vi "const_bias_conductance.vi"() -> ()   [LabVIEW 2010]
uses:
  <vilib>/Utility/file.llb/Write To Spreadsheet File (DBL).vi
  <userlib>/Nanonis Prog Interface V5/Nanonis Prog Interface.lvlib
panel:
  in  "Bias (V)":sgl format="%_5p"
  in  "Feedback?":bool=TRUE
  in  "Settling Time between gate":u32=5
  in  "Wait Time between AVG":i32=1
  out "Input 2 (V)":sgl
  out "XY Graph":cluster{dbl[], dbl[]}(graph)
  in  "Averages":i32=5
  out "Current Gate Voltage (V)":dbl
  in  "Stop":bool
  in  "Increment Gate (V)":dbl
  in  "End Gate (V)":dbl
  in  "Start Gate (V)":dbl
  in  "Filename":string
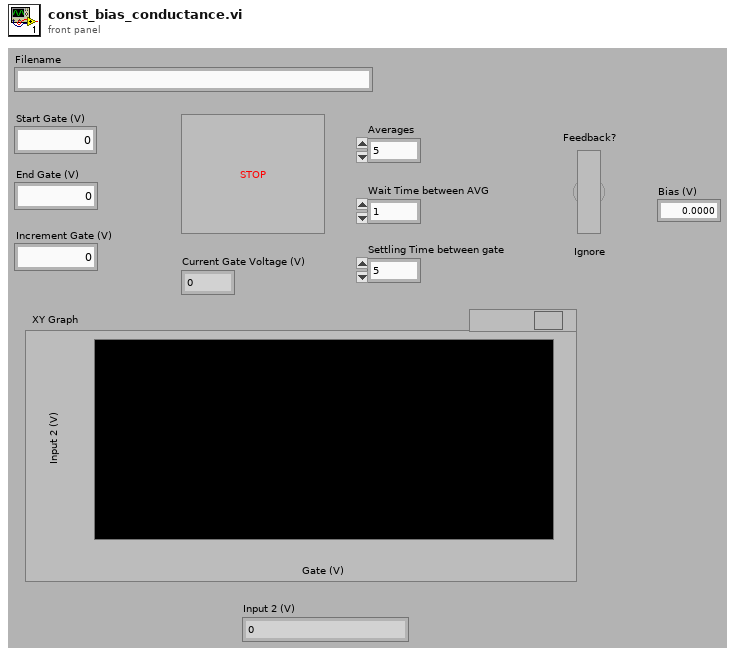
[diagram p1: front panel]
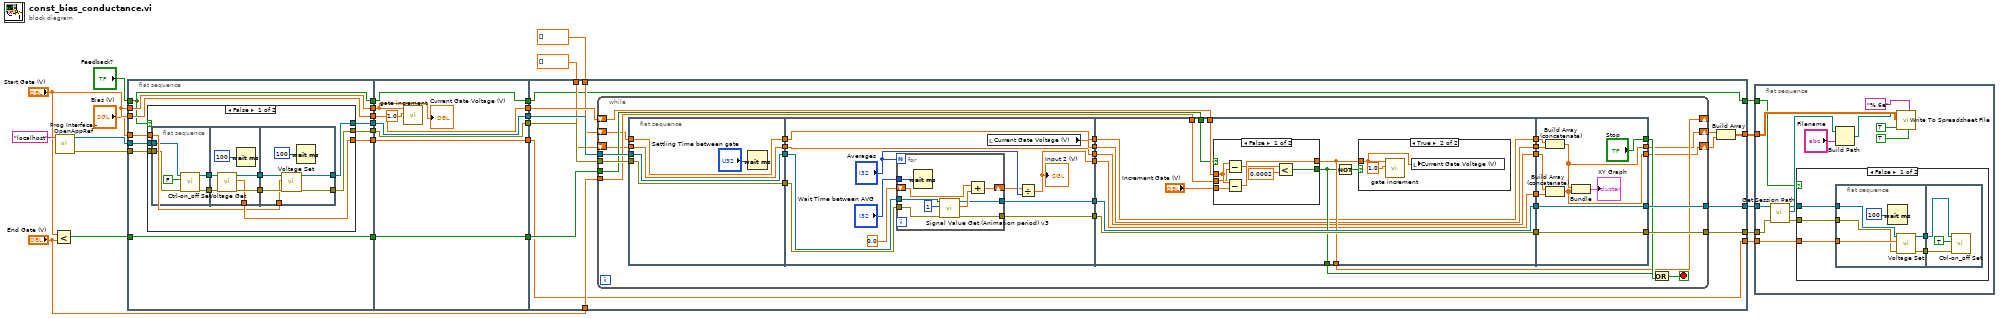
[diagram p0: block diagram]
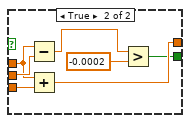
[diagram p4: hidden frame]
diagram:
  n1 = Less?(x="Start Gate (V)", y="End Gate (V)") -> (x < y?=w25:bool)
  n2 = call <userlib>:"Prog Interface - OpenAppRef.vi"("Machine name (local machine IP)"="localhost" ("machine name (localhost)")) -> ("Error out"=w17:errorcluster, "Application reference"=w18:refnum<vi>)  [unwired: 5 in]
  n3 = flat-sequence {
    tunnel: "Start Gate (V)" -> [w36]
    tunnel: "Start Gate (V)" -> [w37]
    tunnel: w25 -> [w38]
    tunnel: w18 -> [w35]
    tunnel: w17 -> [w32]
    tunnel: [w38] -> w13
    tunnel: [w37] -> w12
    tunnel: [w36] -> w11
    tunnel: "Feedback?" -> [w31]
    tunnel: [w34] -> w9
    tunnel: [w33] -> w8
    tunnel: [w31] -> w7
    tunnel: [w30] -> w4
    tunnel: "Bias (V)" -> [w29]
    tunnel: [w76] -> w24
    tunnel: [w75] -> w23
    tunnel: [w74] -> w22
    tunnel: [w73] -> w21
    tunnel: w13 -> [w74]
    tunnel: w12 -> [w73]
    tunnel: w11 -> [w71]
    tunnel: w9 -> [w75]
    tunnel: w8 -> [w76]
    tunnel: w7 -> [w70]
    tunnel: [w70] -> w6
    tunnel: w4 -> [w69]
    tunnel: [w69] -> w3
    tunnel: [w88] -> w27
    tunnel: [w87] -> w26
    tunnel: w24 -> [w90]
    tunnel: w23 -> [w89]
    tunnel: w22 -> [w86]
    tunnel: w21 -> [w85]
    tunnel: "End Gate (V)" -> [w84]
    tunnel: [w81] -> w16
    tunnel: dbl[] [] -> [w80]
    tunnel: dbl[] [] -> [w79]
    tunnel: w6 -> [w78]
    tunnel: [w78] -> w5
    tunnel: w3 -> [w77]
    tunnel: [w77] -> w2
    frame #0 {
      n4 = case shown="False" w31 {
        tunnel: w35 -> [w48 w68]
        tunnel: [w41 w68] -> w34
        tunnel: [w40 w67] -> w33
        tunnel: w32 -> [w47 w67]
        tunnel: [w42 w66] -> w30
        tunnel: w29 -> [w39 w66]
        frame False {
          n5 = flat-sequence {
            tunnel: w48 -> [w53]
            tunnel: w47 -> [w52]
            tunnel: [w50] -> w46
            tunnel: [w49] -> w45
            tunnel: w46 -> [w59]
            tunnel: w45 -> [w58]
            tunnel: [w57] -> w44
            tunnel: [w56] -> w43
            tunnel: [w55] -> w42
            tunnel: w44 -> [w65]
            tunnel: w43 -> [w64]
            tunnel: [w62] -> w41
            tunnel: [w61] -> w40
            tunnel: w39 -> [w60]
            frame #0 {
              n6 = call <userlib>:"Ctrl-on_off Set.vi"("error in (no error)"=w52, "Z Controller ON/OFF"=FALSE, "Application ref in"=w53) -> ("error out"=w49:errorcluster, "Application ref out"=w50:refnum<vi>)  [unwired: 7 in]
            }
            frame #1 {
              n7 = call <userlib>:"Voltage Get.vi"("error in (no error)"=w58, "Application ref in"=w59) -> ("error out"=w57:errorcluster, "Bias (V)"=w55:sgl, "Application ref out"=w56:refnum<vi>)  [unwired: 7 in]
              n8 = Wait (ms)(milliseconds to wait=u32 100) -> ()  [unwired: 1 out]
            }
            frame #2 {
              n9 = call <userlib>:"Voltage Set.vi"("Error in (no error)"=w65, "Bias (V)"=w60, "Application ref in"=w64) -> ("Error out"=w61:errorcluster, "Application ref out"=w62:refnum<vi>)  [unwired: 7 in]
              n10 = Wait (ms)(milliseconds to wait=u32 100) -> ()  [unwired: 1 out]
            }
          }
        }
        frame True {
        }
      }
    }
    frame #1 {
      n11 = call "gate increment.vi"("Increment"=1.0, "Gate Voltage"=w71) -> ()  [unwired: 8 in, 2 out]
      "Current Gate Voltage (V)" <- w71
    }
    frame #2 {
      n12 = while {
        tunnel: w90 -> [w121]
        tunnel: w89 -> [w120]
        tunnel: [w119] -> w88
        tunnel: [w118] -> w87
        tunnel: w86 -> [w107]
        shift-right: [w111] -> _
        shift-left: w85 -> [w109]
        tunnel: w84 -> [w108]
        shift-right: [w101] -> w83
        shift-left: w80 -> [w100]
        shift-right: [w98] -> w82
        shift-left: w79 -> [w93]
        stop <- w112 stop-if-true
        n13 = flat-sequence {
          tunnel: w120 -> [w125]
          tunnel: w121 -> [w126]
          tunnel: [w126] -> w115
          tunnel: [w125] -> w114
          tunnel: w100 -> [w123]
          tunnel: w93 -> [w124]
          tunnel: [w124] -> w94
          tunnel: [w123] -> w92
          tunnel: w115 -> [w138]
          tunnel: w114 -> [w134]
          tunnel: [w133] -> w106
          tunnel: [w132] -> w105
          tunnel: [w131] -> w104
          tunnel: [w129] -> w97
          tunnel: [w130] -> w96
          tunnel: w94 -> [w129]
          tunnel: w92 -> [w128]
          tunnel: [w128] -> w91
          tunnel: [w160] -> w117
          tunnel: [w159] -> w116
          tunnel: [w158] -> w111
          tunnel: [w157] -> w110
          tunnel: w109 -> [w156]
          tunnel: w108 -> [w154]
          tunnel: w107 -> [w153]
          tunnel: w106 -> [w159]
          tunnel: w105 -> [w160]
          tunnel: w104 -> [w151]
          tunnel: [w151] -> w103
          tunnel: [w150] -> w102
          tunnel: [w149] -> w99
          tunnel: w97 -> [w149]
          tunnel: w96 -> [w148]
          tunnel: [w148] -> w95
          tunnel: w91 -> [w150]
          tunnel: [w185] -> w119
          tunnel: [w186] -> w118
          tunnel: w117 -> [w186]
          tunnel: w116 -> [w185]
          tunnel: ["Stop"] -> w113
          tunnel: [w178] -> w101
          tunnel: w103 -> [w183]
          tunnel: w102 -> [w182]
          tunnel: w99 -> [w181]
          tunnel: [w177] -> w98
          tunnel: w95 -> [w180]
          frame #0 {
            n14 = Wait (ms)(milliseconds to wait="Settling Time between gate") -> ()  [unwired: 1 out]
          }
          frame #1 {
            n15 = for {
              N: "Averages" -> [_]
              tunnel: w134 -> [w146]
              tunnel: w138 -> [w145]
              shift-right: [w142] -> w136
              shift-left: sgl 0.0 -> [w143]
              tunnel: [w141] -> w133
              tunnel: [w140] -> w132
              tunnel: "Wait Time between AVG" -> [w139]
              n16 = Wait (ms)(milliseconds to wait=w139) -> ()  [unwired: 1 out]
              n17 = call <userlib>:"Signal Value Get (Animation period) v3.vi"("error in (no error)"=w145, "Signal index (0-127)"=i8 1, "Application ref in"=w146) -> ("error out"=w140:errorcluster, "Signal value"=w144:sgl, "Application ref out"=w141:refnum<vi>)  [unwired: 5 in]
              n18 = Add(x=w143, y=w144) -> (x+y=w142:sgl)
            }
            n19 = local read "Current Gate Voltage (V)"() -> (w131:dbl)
            n20 = Divide(x=w136, y="Averages") -> (x/y=w130:sgl)
            "Input 2 (V)" <- w130
          }
          frame #2 {
            n21 = case shown="False" w153 {
              tunnel: w156 -> [w165 w171]
              tunnel: "Increment Gate (V)" -> [w166 w174]
              tunnel: [w167 w173] -> w158
              tunnel: w154 -> [w164 w172]
              tunnel: [w162 w170] -> w157
              frame False {
                n22 = Subtract(x=w165, y=w164) -> (x-y=w163:dbl)
                n23 = Subtract(x=w165, y=w166) -> (x-y=w167:dbl)
                n24 = Less?(x=w163, y=0.0002) -> (x < y?=w162:bool)
              }
              frame True {
                n25 = Subtract(x=w171, y=w172) -> (x-y=w169:dbl)
                n26 = Add(x=w171, y=w174) -> (x+y=w173:dbl)
                n27 = Greater?(x=w169, y=-0.0002) -> (0:w170:bool)
              }
            }
            n28 = Not(x=w157) -> (.not. x?=w152:bool)
            n29 = case shown="True" w152 {
              tunnel: w158 -> [_ w175]
              frame False {
              }
              frame True {
                n30 = call "gate increment.vi"("Increment"=1.0, "Gate Voltage"=w175) -> ()  [unwired: 8 in, 2 out]
                n31 = local write "Current Gate Voltage (V)"(w175) -> ()
              }
            }
          }
          frame #3 {
            n32 = Build Array (concatenate)(w182, w183) -> (w178:dbl[])
            n33 = Build Array (concatenate)(w181, w180) -> (w177:dbl[])
            n34 = Bundle(w178, w177) -> (→"XY Graph":cluster{dbl[], dbl[]})  [unwired: 1 in]
          }
        }
        n35 = Or(x=w110, y=w113) -> (x .or. y?=w112:bool)
      }
      n36 = Build Array(w83, w82) -> (w81:dbl[][])
    }
  }
  n37 = flat-sequence {
    tunnel: w27 -> [w196]
    tunnel: w26 -> [w195]
    tunnel: w16 -> [w197]
    tunnel: w5 -> [w190]
    tunnel: w2 -> [w189]
    frame #0 {
      n38 = call <userlib>:"Get Session Path.vi"("error in (no error)"=w195, "Application ref in"=w196) -> ("error out"=w187:errorcluster, "Session path"=w192:path, "Application ref out"=w188:refnum<vi>)  [unwired: 7 in]
      n39 = case shown="False" w190 {
        tunnel: w189 -> [w204 _]
        tunnel: w188 -> [w203 _]
        tunnel: w187 -> [w202 _]
        frame False {
          n40 = flat-sequence {
            tunnel: w204 -> [w210]
            tunnel: w203 -> [w209]
            tunnel: w202 -> [w208]
            tunnel: [w207] -> w201
            tunnel: [w206] -> w200
            tunnel: w201 -> [w213]
            tunnel: w200 -> [w212]
            frame #0 {
              n41 = Wait (ms)(milliseconds to wait=u32 100) -> ()  [unwired: 1 out]
              n42 = call <userlib>:"Voltage Set.vi"("Error in (no error)"=w208, "Bias (V)"=w210, "Application ref in"=w209) -> ("Error out"=w206:errorcluster, "Application ref out"=w207:refnum<vi>)  [unwired: 7 in]
            }
            frame #1 {
              n43 = call <userlib>:"Ctrl-on_off Set.vi"("error in (no error)"=w212, "Z Controller ON/OFF"=TRUE, "Application ref in"=w213) -> ()  [unwired: 7 in, 2 out]
            }
          }
        }
        frame True {
        }
      }
      n44 = Build Path(base path=w192, name or relative path="Filename") -> (appended path=w194:path)
      n45 = call-poly <vilib>:"Write To Spreadsheet File.vi"("transpose? (no:F)"=TRUE ("append to file? (new file:F)"), "format (%.3f)"="%.6e", "append to file? (new file:F)"=TRUE, "2D data"=w197, "file path (dialog if empty)"=w194) -> ()  [unwired: 3 in, 1 out]
    }
  }
